vi "CalcStones.vi"(9 "StoneNumber":u64, 10 "BlinkNumber(n-0)":i32, 11 "DataIn":map{cluster{"Number":u64, "Blinks":i32}, u64}(c390)) -> (2 "NumberOfStones":u64, 3 "DataOut":map{cluster{"Number":u64, "Blinks":i32}, u64}(c390))   [LabVIEW 2023, in "2024_11.lvclass"]
uses:
  2024_11.lvclass
  2024_11.lvclass/2024_11.ctl
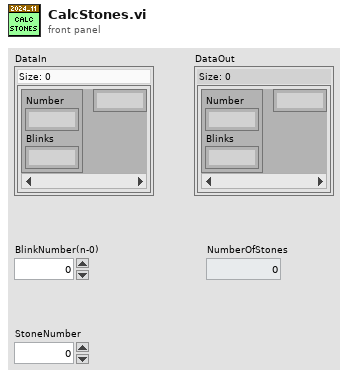
[diagram p1: front panel]
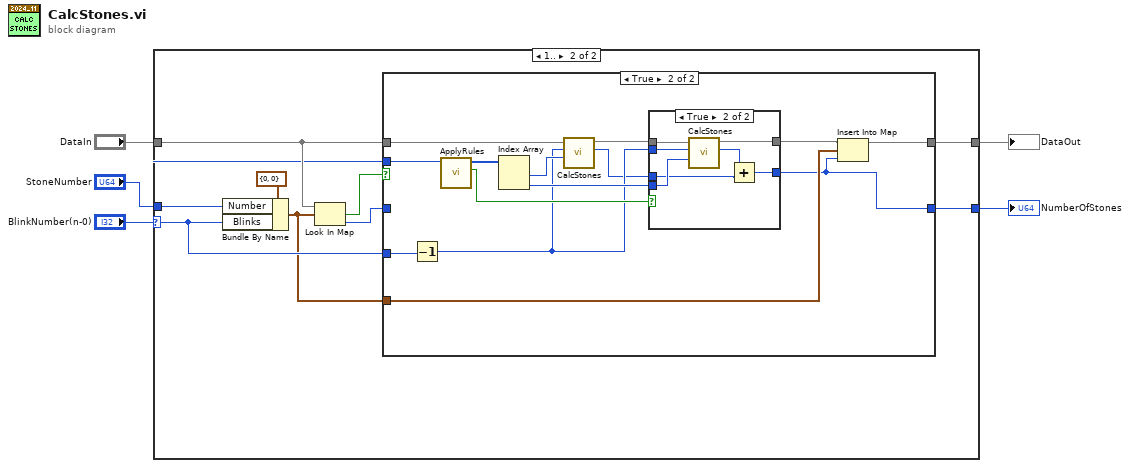
[diagram p0: block diagram]
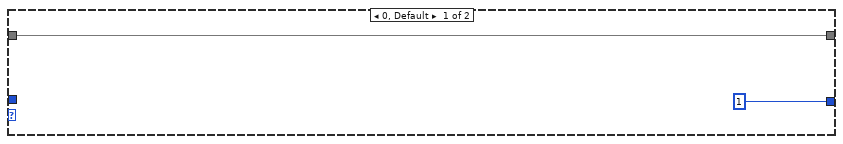
[diagram p2: hidden frame]
diagram:
  n1 = case shown="1.." "BlinkNumber(n-0)" {
    selector: "BlinkNumber(n-0)" -> [_ w9]
    tunnel: "DataIn" -> [w7 w13]
    tunnel: [w7 w12] -> w4
    tunnel: [1 ("value") w11] -> w3
    tunnel: "StoneNumber" -> [_ w10]
    frame 0, Default {
    }
    frame 1.. {
      n2 = Bundle By Name(cluster=cluster{"Number":u64, "Blinks":i32} {"Number"=0, "Blinks"=0} ("key"), "Number"=w10, "Blinks"=w9) -> (w8:cluster{"Number":u64, "Blinks":i32})
      n3 = Look In Map(map=w13, key=w8) -> (key not found?=w15:bool, value=w14:u64)  [unwired: 1 in]
      n4 = case shown="True" w15 {
        tunnel: w14 -> [w18 _]
        tunnel: [w18 w19] -> w11
        tunnel: [w17 w21] -> w12
        tunnel: w13 -> [w17 w27]
        tunnel: w10 -> [_ w32]
        tunnel: w9 -> [_ w31]
        tunnel: w8 -> [_ w20]
        frame False {
        }
        frame True {
          n5 = Decrement(x=w31) -> (x-1=w24:i32)
          n6 = call "ApplyRules.vi"("Numeric"=w32) -> ("StoneSplit"=w29:bool, "Array"=w30:u64[])  [unwired: 9 in]
          n7 = Index Array(array=w30) -> (element #1=w25:u64, element #2=w28:u64)  [unwired: 2 in]
          n8 = call "CalcStones.vi"("StoneNumber"=w25, "BlinkNumber(n-0)"=w24, "DataIn"=w27) -> ("NumberOfStones"=w23:u64, "DataOut"=w26:map{cluster{"Number":u64, "Blinks":i32}, u64})  [unwired: 7 in]
          n9 = case shown="True" w29 {
            tunnel: w26 -> [w33 w41]
            tunnel: [w33 w40] -> w22
            tunnel: w24 -> [_ w39]
            tunnel: w28 -> [_ w38]
            tunnel: w23 -> [w34 w36]
            tunnel: [w34 w35] -> w19
            frame False {
            }
            frame True {
              n10 = call "CalcStones.vi"("StoneNumber"=w38, "BlinkNumber(n-0)"=w39, "DataIn"=w41) -> ("NumberOfStones"=w37:u64, "DataOut"=w40:map{cluster{"Number":u64, "Blinks":i32}, u64})  [unwired: 7 in]
              n11 = Add(x=w37, y=w36) -> (x+y=w35:u64)
            }
          }
          n12 = Insert Into Map(map in=w22, key=w20, value=w19) -> (map out=w21:map{cluster{"Number":u64, "Blinks":i32}, u64})  [unwired: 2 out]
        }
      }
    }
  }
  "NumberOfStones" <- w3
  "DataOut" <- w4
